vi "状态参数解析.vi"(8 "error in (no error)":errorcluster caption="错误输入（无错误）", 11 "字符串":string) -> (0 "error out":errorcluster caption="错误输出", 3 "簇":T1 {"仪器时间" format="%<%Y/%m/%d %H:%M:%S>T"; "门状态" items=["关闭", "打开"]; "采样模式" items=["定时留样"=1, "时间等比"=2, "同步留样"=3, "外控留样"=4, "超标留样"=5]; "工作进程" items=["停止中", "启动延时", "外置泵延时", "管路润洗", "管存", "留样", "出水管路排空", "采水管路排空"]; "工作状态" items=["停止", "运行"]})   [LabVIEW 2016, in "德润超标留样.lvlib"]
panel:
  out "仪器时间1111":string
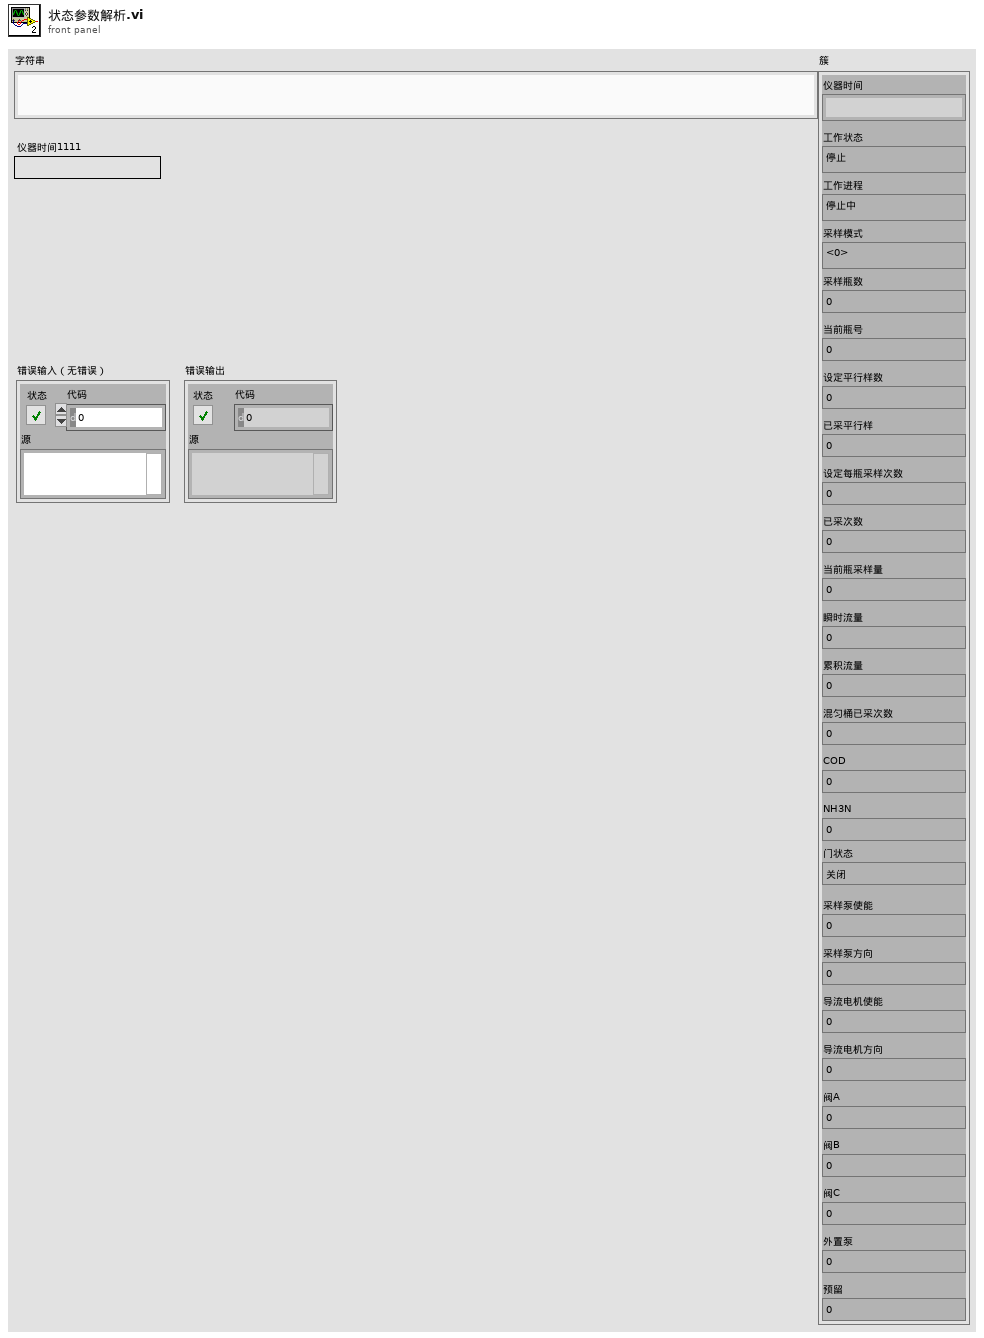
[diagram p1: front panel]
types:
  T1 = cluster{"仪器时间":timestamp, "工作状态":u16, "工作进程":u16, "采样模式":u16, "采样瓶数":dbl, "当前瓶号":dbl, "设定平行样数":dbl, "已采平行样":dbl, "设定每瓶采样次数":dbl, "已采次数":dbl, "当前瓶采样量":dbl, "瞬时流量":dbl, "累积流量":dbl, "混匀桶已采次数":dbl, "COD":dbl, "NH3N":dbl, "门状态":u16, "采样泵使能":dbl, "采样泵方向":dbl, "导流电机使能":dbl, "导流电机方向":dbl, "阀A":dbl, "阀B":dbl, "阀C":dbl, "外置泵":dbl, "预留":dbl}
  T2 = typedef "LVDateTimeRec.ctl" = cluster{"秒数的小数部分":dbl, "秒":i32, "分":i32, "时":i32, "日":i32, "月":i32, "年":i32, "天数（周）":i32, "天数（年）":i32, "DST":i32}
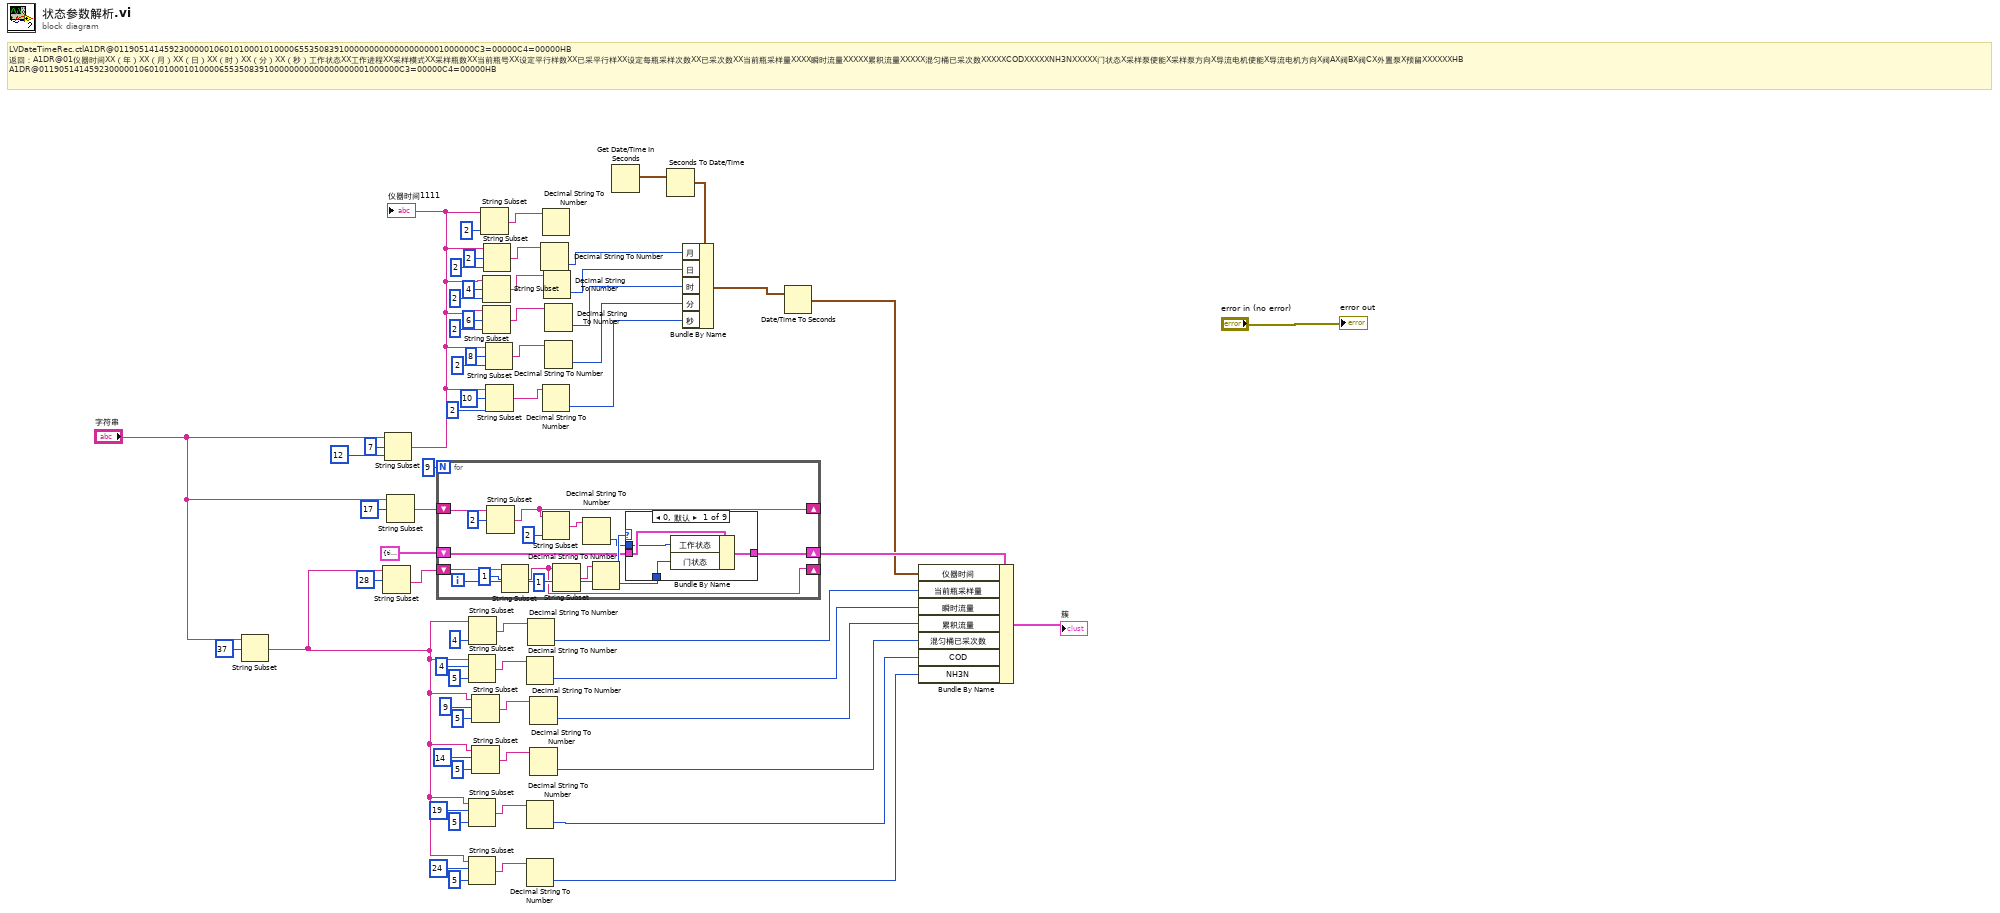
[diagram p0: block diagram]
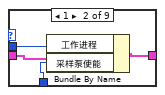
[diagram p2: hidden frame]
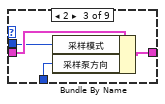
[diagram p3: hidden frame]
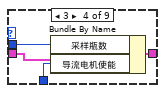
[diagram p4: hidden frame]
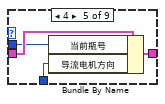
[diagram p5: hidden frame]
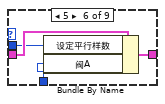
[diagram p6: hidden frame]
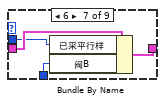
[diagram p7: hidden frame]
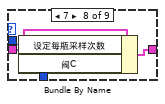
[diagram p8: hidden frame]
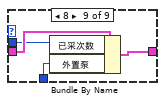
[diagram p9: hidden frame]
diagram:
  # "LVDateTimeRec.ctlA1DR@011905141459230000010601010001010000655350839100000000000000000001000000C3=00000C4=00000HB\n返回：A1DR@01仪器时间XX（年）XX（月）XX（日）XX（时）XX（分）XX（秒）工作状态XX工作进程XX采样模式XX采样瓶数XX当前瓶号XX设定平行样数XX已采平行样XX设定每瓶采样次数XX已采次数XX当前瓶采样量XXXX瞬时流量XXXXX累积流量XXXXX混匀桶已采次数XXXXXCODXXXXXNH3NXXXXX门状态X采样泵使能X采样泵方向X导流电机使能X导流电机方向X阀AX阀BX阀CX外置泵X预留XXXXXXHB\nA1DR@011905141459230000010601010001010000655350839100000000000000000001000000C3=00000C4=00000HB"
  n1 = String Subset(string="字符串", offset (0)=37 ("偏移量(0)")) -> (substring=w4:string)  [unwired: 1 in]
  n2 = String Subset(string=w4, offset (0)=28 ("偏移量(0)")) -> (substring=w5:string)  [unwired: 1 in]
  n3 = String Subset(string="字符串", offset (0)=7 ("偏移量(0)"), length (rest)=12 ("长度（剩余）")) -> (substring=w43:string)
  "仪器时间1111" <- w43
  n4 = String Subset(string="字符串", offset (0)=17 ("偏移量(0)")) -> (substring=w58:string)  [unwired: 1 in]
  n5 = for {
    N: 9 -> [_]
    shift-right: [w77] -> _
    shift-left: w58 -> [w79]
    shift-right: [w71] -> w57
    shift-left: T1 {"仪器时间"=timestamp(0 s since 1904-01-01), "工作状态"=0, "工作进程"=0, "采样模式"=1, "采样瓶数"=6.0, "当前瓶号"=1.0, "设定平行样数"=1.0, "已采平行样"=0.0, "设定每瓶采样次数"=1.0, "已采次数"=1.0, "当前瓶采样量"=0.0, "瞬时流量"=0.0, "累积流量"=0.0, "混匀桶已采次数"=0.0, "COD"=0.0, "NH3N"=0.0, "门状态"=0, "采样泵使能"=0.0, "采样泵方向"=0.0, "导流电机使能"=0.0, "导流电机方向"=0.0, "阀A"=0.0, "阀B"=0.0, "阀C"=0.0, "外置泵"=0.0, "预留"=0.0} ("簇") -> [w73]
    shift-right: [w65] -> _
    shift-left: w5 -> [w69]
    i -> [w75]
    n6 = String Subset(string=w79, offset (0)=2 ("偏移量(0)")) -> (substring=w77:string)  [unwired: 1 in]
    n7 = String Subset(string=w69, offset (0)=1 ("偏移量(0)")) -> (substring=w65:string)  [unwired: 1 in]
    n8 = String Subset(string=w77, length (rest)=2 ("长度（剩余）")) -> (substring=w74:string)  [unwired: 1 in]
    n9 = String Subset(string=w65, length (rest)=1 ("长度（剩余）")) -> (substring=w67:string)  [unwired: 1 in]
    n10 = Decimal String To Number(string=w74) -> (number=w72:i32)  [unwired: 2 in, 1 out]
    n11 = Decimal String To Number(string=w67) -> (number=w66:i32)  [unwired: 2 in, 1 out]
    n12 = case shown="0, 默认" w75 {
      tunnel: w73 -> [w83 w85 w91 w94 w99 w103 w107 w111 w115]
      tunnel: w72 -> [w82 w87 w90 w95 w98 w102 w106 w110 w114]
      tunnel: [w81 w86 w89 w93 w97 w101 w105 w109 w113] -> w71
      tunnel: w66 -> [w80 w84 w88 w92 w96 w100 w104 w108 w112]
      frame 0, Default {
        n13 = Bundle By Name(cluster=w83, "工作状态"=w82, "门状态"=w80) -> (w81:T1)
      }
      frame 1 {
        n14 = Bundle By Name(cluster=w85, "工作进程"=w87, "采样泵使能"=w84) -> (w86:T1)
      }
      frame 2 {
        n15 = Bundle By Name(cluster=w91, "采样模式"=w90, "采样泵方向"=w88) -> (w89:T1)
      }
      frame 3 {
        n16 = Bundle By Name(cluster=w94, "采样瓶数"=w95, "导流电机使能"=w92) -> (w93:T1)
      }
      frame 4 {
        n17 = Bundle By Name(cluster=w99, "当前瓶号"=w98, "导流电机方向"=w96) -> (w97:T1)
      }
      frame 5 {
        n18 = Bundle By Name(cluster=w103, "设定平行样数"=w102, "阀A"=w100) -> (w101:T1)
      }
      frame 6 {
        n19 = Bundle By Name(cluster=w107, "已采平行样"=w106, "阀B"=w104) -> (w105:T1)
      }
      frame 7 {
        n20 = Bundle By Name(cluster=w111, "设定每瓶采样次数"=w110, "阀C"=w108) -> (w109:T1)
      }
      frame 8 {
        n21 = Bundle By Name(cluster=w115, "已采次数"=w114, "外置泵"=w112) -> (w113:T1)
      }
    }
  }
  n22 = String Subset(string=w4, offset (0)=4 ("偏移量(0)"), length (rest)=5 ("长度（剩余）")) -> (substring=w29:string)
  n23 = String Subset(string=w4, offset (0)=19 ("偏移量(0)"), length (rest)=5 ("长度（剩余）")) -> (substring=w16:string)
  n24 = String Subset(string=w4, offset (0)=24 ("偏移量(0)"), length (rest)=5 ("长度（剩余）")) -> (substring=w10:string)
  n25 = String Subset(string=w4, length (rest)=4 ("长度（剩余）")) -> (substring=w31:string)  [unwired: 1 in]
  n26 = String Subset(string=w4, offset (0)=9 ("偏移量(0)"), length (rest)=5 ("长度（剩余）")) -> (substring=w23:string)
  n27 = String Subset(string=w4, offset (0)=14 ("偏移量(0)"), length (rest)=5 ("长度（剩余）")) -> (substring=w21:string)
  n28 = String Subset(string=w43, length (rest)=2 ("长度（剩余）")) -> (substring=w1:string)  [unwired: 1 in]
  n29 = String Subset(string=w43, offset (0)=4 ("偏移量(0)"), length (rest)=2 ("长度（剩余）")) -> (substring=w47:string)
  n30 = String Subset(string=w43, offset (0)=6 ("偏移量(0)"), length (rest)=2 ("长度（剩余）")) -> (substring=w36:string)
  n31 = String Subset(string=w43, offset (0)=2 ("偏移量(0)"), length (rest)=2 ("长度（剩余）")) -> (substring=w51:string)
  n32 = String Subset(string=w43, offset (0)=8 ("偏移量(0)"), length (rest)=2 ("长度（剩余）")) -> (substring=w37:string)
  n33 = String Subset(string=w43, offset (0)=10 ("偏移量(0)"), length (rest)=2 ("长度（剩余）")) -> (substring=w38:string)
  n34 = Decimal String To Number(string=w29) -> (number=w26:i32)  [unwired: 2 in, 1 out]
  n35 = Decimal String To Number(string=w16) -> (number=w12:i32)  [unwired: 2 in, 1 out]
  n36 = Decimal String To Number(string=w10) -> (number=w11:i32)  [unwired: 2 in, 1 out]
  n37 = Decimal String To Number(string=w31) -> (number=w30:i32)  [unwired: 2 in, 1 out]
  n38 = Decimal String To Number(string=w23) -> (number=w22:i32)  [unwired: 2 in, 1 out]
  n39 = Decimal String To Number(string=w21) -> (number=w13:i32)  [unwired: 2 in, 1 out]
  n40 = Decimal String To Number(string=w51) -> (number=w50:i32)  [unwired: 2 in, 1 out]
  n41 = Decimal String To Number(string=w1) -> ()  [unwired: 2 in, 2 out]
  n42 = Decimal String To Number(string=w38) -> (number=w33:i32)  [unwired: 2 in, 1 out]
  n43 = Decimal String To Number(string=w47) -> (number=w46:i32)  [unwired: 2 in, 1 out]
  n44 = Decimal String To Number(string=w36) -> (number=w35:i32)  [unwired: 2 in, 1 out]
  n45 = Decimal String To Number(string=w37) -> (number=w34:i32)  [unwired: 2 in, 1 out]
  n46 = Get Date/Time In Seconds() -> (seconds since 1Jan1904=w3:timestamp)
  n47 = Seconds To Date/Time(time stamp (now)=w3) -> (date time rec=w2:T2)  [unwired: 1 in]
  n48 = Bundle By Name(cluster=w2, "月"=w50, "日"=w46, "时"=w35, "分"=w34, "秒"=w33) -> (w56:T2)
  n49 = Date/Time To Seconds(2:w56) -> (0:w55:timestamp)  [unwired: 1 in]
  n50 = Bundle By Name(cluster=w57, "仪器时间"=w55, "当前瓶采样量"=w30, "瞬时流量"=w26, "累积流量"=w22, "混匀桶已采次数"=w13, "COD"=w12, "NH3N"=w11) -> (→"簇":T1)
  "error out" <- "error in (no error)"
